vi "ExitChannelSettings.vi"(8 "error in (no error)":errorcluster) -> (0 "error out":errorcluster, 3 "Confirmed":bool)   [LabVIEW 2019]
panel:
  in  "Btn-Cancel":bool
  in  "Btn-OK":bool
  # "You are exiting without saving your settings changes.\n\nDo you want to save?"
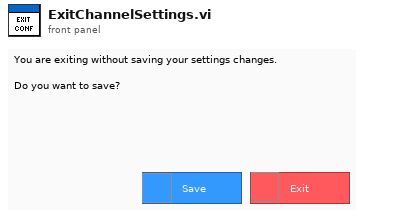
[diagram p1: front panel]
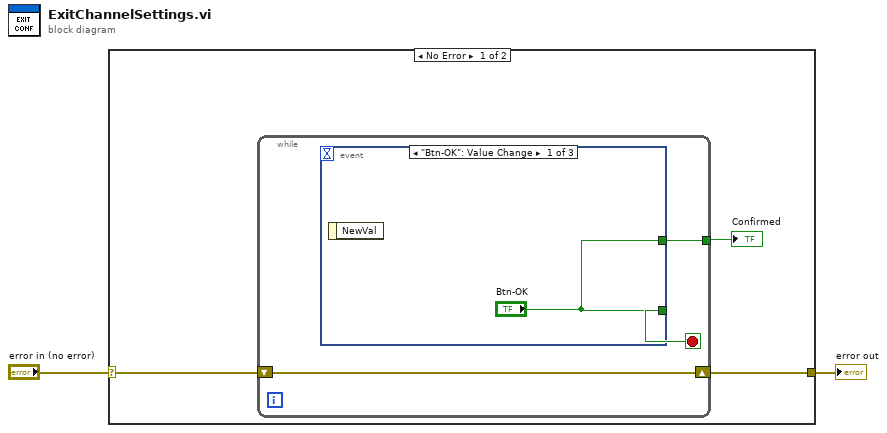
[diagram p0: block diagram]
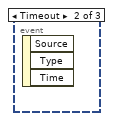
[diagram p2: hidden frame]
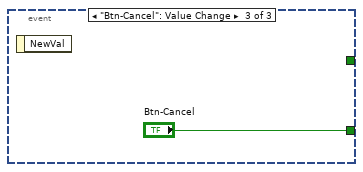
[diagram p3: hidden frame]
diagram:
  n1 = case shown="No Error" "error in (no error)" {
    selector: "error in (no error)" -> [w3 w11]
    tunnel: [w4 w11] -> w1
    frame No Error {
      n2 = while {
        tunnel: [w7] -> w5
        shift-right: [w6] -> w4
        shift-left: w3 -> [w6]
        stop <- w8 stop-if-true
        n3 = event shown="[0] \"Btn-OK\": Value Change" {
          selector: _ -> [_ _ _]
          dyn-events: _ -> [_ _ _]
          timeout: _ -> [_ _ _]
          tunnel: ["Btn-OK" _ "Btn-Cancel"] -> w8
          tunnel: ["Btn-OK" _ _] -> w7
          event "Btn-OK": Value Change {
            n4 = event-data() -> ()  [unwired: 1 in, 1 out]
          }
          event Timeout {
            n5 = event-data() -> ()  [unwired: 1 in, 3 out]
          }
          event "Btn-Cancel": Value Change {
            n6 = event-data() -> ()  [unwired: 1 in, 1 out]
          }
        }
      }
      "Confirmed" <- w5
    }
    frame Error {
    }
  }
  "error out" <- w1
